vi "AlliGator Load Calibration Phasor Series.vi"(8 "Error In":errorcluster, 10 "File Path":path, 11 "Calibration Phasor Series in":T1={"m Array"=[], "phi Array"=[], "Phasor Frequency"=80000000.0, "Calibration Lifetime"=1e-09}) -> (0 "error out":errorcluster, 1 "Phasor Frequency":dbl[unit], 2 "XML File Path":path, 3 "Calibration Phasor Series out":T1={"m Array"=[], "phi Array"=[], "Phasor Frequency"=80000000.0, "Calibration Lifetime"=1e-09}, 4 "Message":string)   [LabVIEW 2021, in "AlliGator Phasor Calibration.lvlib"]
doc: "Loads <B>Phasor Calibration Series</B>."
uses:
  AlliGator Phasor Calibration.lvlib
  Phasor/Phasor Reference Series.ctl
  e60497df-e62f-4827-a05e-c8d2655a0395.vi
  e60497df-e62f-4827-a05e-c8d2655a0395.vi/8a80743f-1319-44c8-96b0-3ef8fc688731.vi
  e60497df-e62f-4827-a05e-c8d2655a0395.vi/931f4f8f-d8c6-4056-833f-5c8fe97b24b9.vi
  <vilib>/Utility/error.llb/Error Cluster From Error Code.vi
  <vilib>/ErrorRing/Error Ring.xnode
  Files/Files.lvlib
  Settings/AlliGator Settings.lvlib
  Phasor/Phasor.lvlib
panel:
  # "see the AlliGator License on the block diagram (Ctrl+E or Window:Show Block Diagram)"
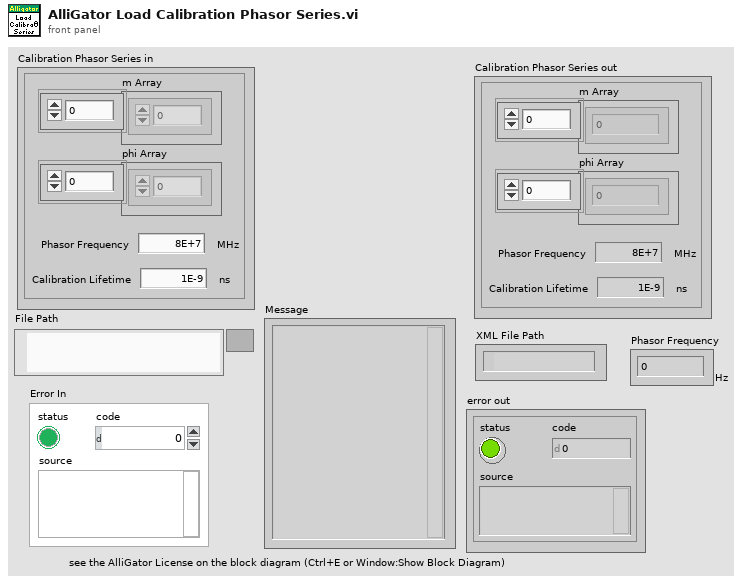
[diagram p1: front panel]
types:
  T1 = typedef "Phasor.lvlib/Phasor Reference Series.ctl" = cluster{"m Array":dbl[], "phi Array":dbl[], "Phasor Frequency":dbl[unit], "Calibration Lifetime":dbl[unit]}
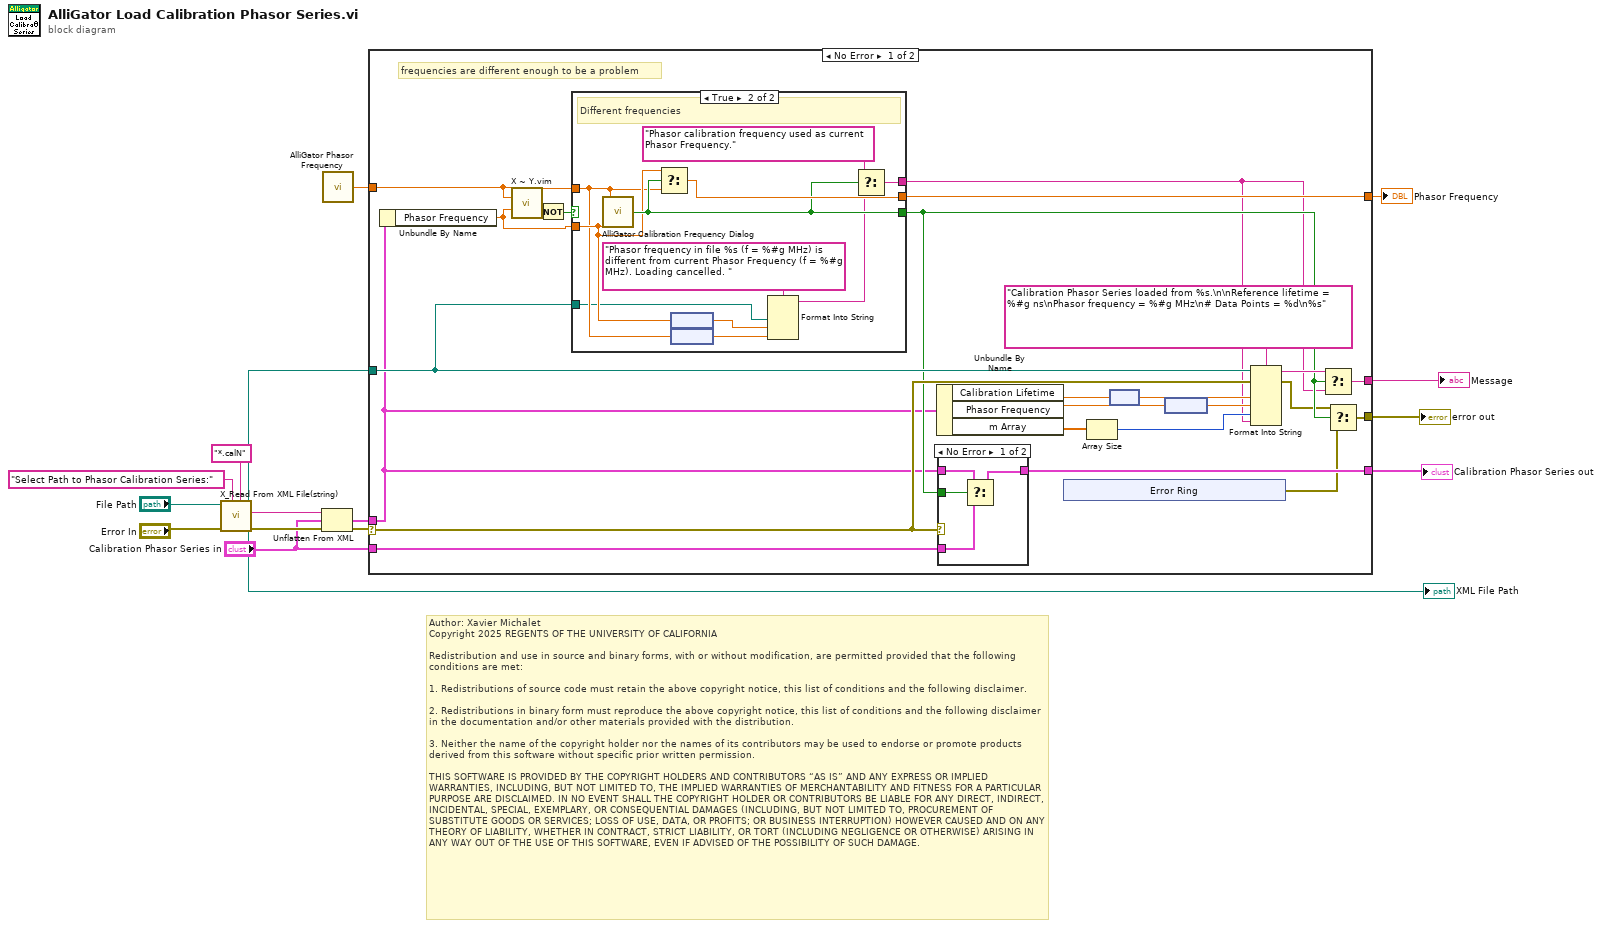
[diagram p0: block diagram]
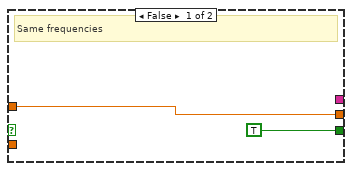
[diagram p3: hidden frame]
diagram:
  # "Author: Xavier Michalet\nCopyright 2025 REGENTS OF THE UNIVERSITY OF CALIFORNIA\n\nRedistribution and use in source and binary forms, with or without modification, are permitted provided that the following conditions are met:\n\n1. Redistributions of source code must retain the above copyright notice, this list of conditions and the following disclaimer.\n\n2. Redistributions in binary form must reproduce the above copyright notice, this list of conditions and the following disclaimer in the documentation and/or other materials provided with the distribution.\n\n3. Neither the name of the copyright holder nor the names of its contributors may be used to endorse or promote products derived from this software without specific prior written permission.\n\nTHIS SOFTWARE IS PROVIDED BY THE COPYRIGHT HOLDERS AND CONTRIBUTORS “AS IS” AND ANY EXPRESS OR IMPLIED WARRANTIES, INCLUDING, BUT NOT LIMITED TO, THE IMPLIED WARRANTIES OF MERCHANTABILITY AND FITNESS FOR A PARTICULAR PURPOSE ARE DISCLAIMED. IN NO EVENT SHALL THE COPYRIGHT HOLDER OR CONTRIBUTORS BE LIABLE FOR ANY DIRECT, INDIRECT, INCIDENTAL, SPECIAL, EXEMPLARY, OR CONSEQUENTIAL DAMAGES (INCLUDING, BUT NOT LIMITED TO, PROCUREMENT OF SUBSTITUTE GOODS OR SERVICES; LOSS OF USE, DATA, OR PROFITS; OR BUSINESS INTERRUPTION) HOWEVER CAUSED AND ON ANY THEORY OF LIABILITY, WHETHER IN CONTRACT, STRICT LIABILITY, OR TORT (INCLUDING NEGLIGENCE OR OTHERWISE) ARISING IN ANY WAY OUT OF THE USE OF THIS SOFTWARE, EVEN IF ADVISED OF THE POSSIBILITY OF SUCH DAMAGE."
  n1 = call "X_Read From XML File(string).vi"("pattern (*.xml)"="*.calN", "Prompt"="Select Path to Phasor Calibration Series:", "error in (no error)"="Error In", "XML File Path"="File Path") -> ("error out"=w15:errorcluster, "XML Elements"=w14:string, "XML File Path(duplicate)"=w3:path)  [unwired: 5 in]
  "XML File Path" <- w3
  n2 = Unflatten From XML(xml string=w14, type="Calibration Phasor Series in", error in (no error)=w15) -> (value=w8:T1, error out=w9:errorcluster)
  n3 = call "AlliGator Phasor Frequency.vi"() -> ("Phasor Frequency"=w2:dbl[unit])
  n4 = case shown="No Error" w9 {
    selector: w9 -> [w32 w64]
    tunnel: [w38 w63] -> w6
    tunnel: "Calibration Phasor Series in" -> [w29 w63]
    tunnel: [w27 _] -> w4
    tunnel: w3 -> [w26 _]
    tunnel: [w25 w62] -> w1
    tunnel: [w22 w64] -> w5
    tunnel: w2 -> [w20 w62]
    tunnel: w8 -> [w19 _]
    frame No Error {
      # "frequencies are different enough to be a problem"
      n5 = Unbundle By Name(w19) -> ("Phasor Frequency"=w30:dbl[unit])
      n6 = call "X ~ Y.vim"("X"=w20, "Y"=w30) -> ("X ~= Y?"=w39:bool)  [unwired: 13 in]
      n7 = Not(x=w39) -> (.not. x?=w31:bool)
      n8 = case shown="True" w31 {
        tunnel: w20 -> [w50 w53]
        tunnel: w30 -> [_ w55]
        tunnel: [TRUE ("Use Calibration Frequency?") w59] -> w24
        tunnel: [w50 w61] -> w25
        tunnel: [_ w58] -> w16
        tunnel: w26 -> [_ w51]
        frame False {
          # "Same frequencies"
        }
        frame True {
          # "Different frequencies"
          n9 = call "AlliGator Calibration Frequency Dialog.vi"("Calibration Phasor Frequency"=w55, "Internal Phasor Frequency"=w53) -> ("Use Calibration Frequency?"=w59:bool)
          n10 = Select(t=w55, s=w59, f=w53) -> (s? t:f=w61:dbl[unit])
          n11 = node(w55) -> (w57:dbl)
          n12 = node(w53) -> (w54:dbl)
          n13 = Format Into String(format string="Phasor frequency in file %s (f = %#g MHz) is different from current Phasor Frequency (f = %#g MHz). Loading cancelled. ", w51, w57, w54) -> (resulting string=w52:string)  [unwired: 2 in, 1 out]
          n14 = Select(t="Phasor calibration frequency used as current Phasor Frequency." ("format string"), s=w59, f=w52) -> (s? t:f=w58:string)
        }
      }
      n15 = Unbundle By Name(w19) -> ("Calibration Lifetime"=w37:dbl[unit], "Phasor Frequency"=w36:dbl[unit], "m Array"=w18:dbl[])
      n16 = case shown="No Error" w32 {
        tunnel: w19 -> [w46 w48]
        tunnel: [w44 w48] -> w38
        tunnel: w29 -> [w45 _]
        tunnel: w24 -> [w47 _]
        frame No Error {
          n17 = Select(t=w46, s=w47, f=w45) -> (s? t:f=w44:T1)
        }
        frame Error {
        }
      }
      n18 = xnode "Error Ring"() -> ("error out"=w21:errorcluster)
      n19 = Array Size(array=w18) -> (size(s)=w17:i32)
      n20 = node(w37) -> (w35:dbl)
      n21 = node(w36) -> (w34:dbl)
      n22 = Format Into String(format string="Calibration Phasor Series loaded from %s.\n\nReference lifetime = %#g ns\nPhasor frequency = %#g MHz\n# Data Points = %d\n%s", error in=w32, w26, w35, w34, w17, w16) -> (resulting string=w28:string, error out=w23:errorcluster)  [unwired: 1 in]
      n23 = Select(t=w28, s=w24, f=w16) -> (s? t:f=w27:string)
      n24 = Select(t=w23, s=w24, f=w21) -> (s? t:f=w22:errorcluster)
    }
    frame Error {
    }
  }
  "Calibration Phasor Series out" <- w6
  "error out" <- w5
  "Message" <- w4
  "Phasor Frequency" <- w1
